vi "dd2.vi"(8 "error in":errorcluster, 11 "Class 11 in":refnum<class "Class 11.lvclass">) -> (0 "error out":errorcluster, 3 "Class 11 out":refnum<class "Class 11.lvclass">)   [LabVIEW 2026, in "Untitled Library 1.lvlib" / "Class 11.lvclass"]
uses:
  Class 11.lvclass
  Class 11.lvclass/Class 11.ctl
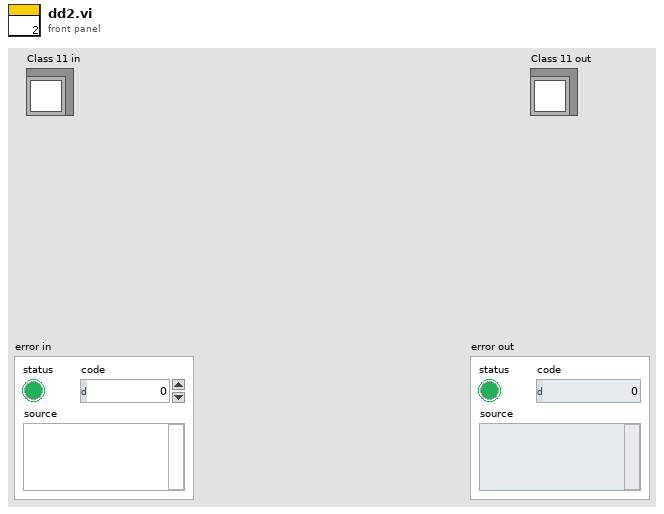
[diagram p1: front panel]
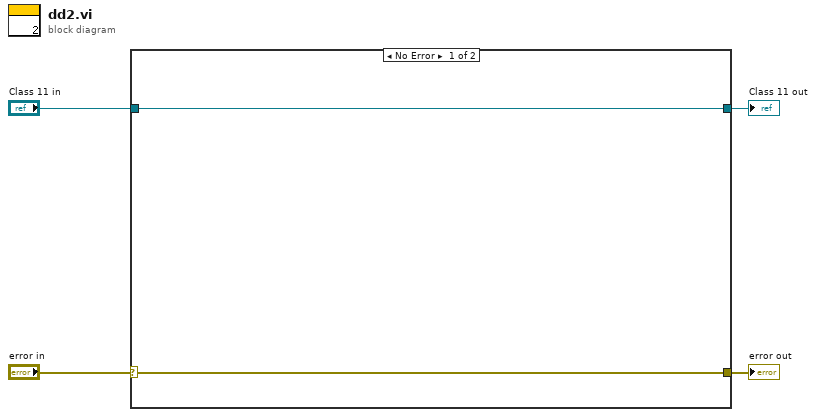
[diagram p0: block diagram]
diagram:
  n1 = case shown="No Error" "error in" {
    selector: "error in" -> [w5 w8]
    tunnel: [w5 w8] -> w1
    tunnel: [w6 w7] -> w3
    tunnel: "Class 11 in" -> [w6 w7]
    frame No Error {
    }
    frame Error {
    }
  }
  "Class 11 out" <- w3
  "error out" <- w1
